vi "LINC Common Command Handler.vi"(6 "GUID":string, 8 "error in (no error)":errorcluster, 9 "command data in":string, 10 "command name in":string, 11 "LINC session":refnum<class "LINC.lvclass">) -> (0 "error out":errorcluster, 2 "application command":bool, 3 "dup LINC session":refnum<class "LINC.lvclass">)   [LabVIEW 2018, in "STEPkgDriver_LINC.lvlib" / "LINC.lvclass"]
uses:
  LINC.lvclass
  STEPkgDriver_LINC.lvlib
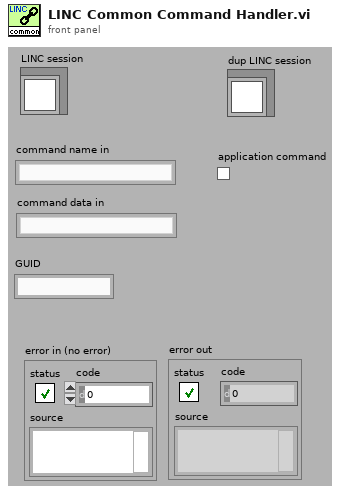
[diagram p1: front panel]
types:
  T1 = enum32{"Invalid", "Standard", "Closed", "Hidden", "Minimized", "Maximized"}
  T2 = cluster{"vi":string, "control":string, "value":variant}
  T3 = cluster{"mode (NO_SIM)":enum16{"NO_SIM", "SIM_EN", "SIM_DS"}, "defer update (F)":bool}
  T4 = typedef "LVRectTypeDef.ctl" = cluster{"Left":i16, "Top":i16, "Right":i16, "Bottom":i16}
  T5 = cluster{"VI":string, "CONTROL":string, "I16":i16}
  T6 = cluster{"VI":string, "CONTROL":string, "I32":i32}
  T7 = cluster{"VI":string, "CONTROL":string, "I64":i64}
  T8 = cluster{"VI":string, "CONTROL":string, "U16":u16}
  T9 = cluster{"VI":string, "CONTROL":string, "U32":u32}
  T10 = cluster{"VI":string, "CONTROL":string, "U64":u64}
  T11 = cluster{"VI":string, "CONTROL":string, "SGL":sgl}
  T12 = cluster{"VI":string, "CONTROL":string, "DBL":dbl}
  T13 = cluster{"VI":string, "CONTROL":string, "BOOL":bool}
  T14 = cluster{"VI":string, "CONTROL":string, "STR":string}
  T15 = cluster{"VI":string, "CONTROL":string, "PATH":string}
  T16 = cluster{"PACKET":string, "ITEM":string, "ST":bool, "VAL":i8}
  T17 = cluster{"PACKET":string, "ITEM":string, "ST":bool, "VAL":i16}
  T18 = cluster{"PACKET":string, "ITEM":string, "ST":bool, "VAL":i32}
  T19 = cluster{"PACKET":string, "ITEM":string, "ST":bool, "VAL":i64}
  T20 = cluster{"PACKET":string, "ITEM":string, "ST":bool, "VAL":u8}
  T21 = cluster{"PACKET":string, "ITEM":string, "ST":bool, "VAL":u16}
  T22 = cluster{"PACKET":string, "ITEM":string, "ST":bool, "VAL":u32}
  T23 = cluster{"PACKET":string, "ITEM":string, "ST":bool, "VAL":u64}
  T24 = cluster{"PACKET":string, "ITEM":string, "ST":bool, "VAL":sgl}
  T25 = cluster{"PACKET":string, "ITEM":string, "ST":bool, "VAL":dbl}
  T26 = cluster{"PACKET":string, "ITEM":string, "ST":bool, "VAL":bool}
  T27 = cluster{"PACKET":string, "ITEM":string, "ST":bool, "VAL":string}
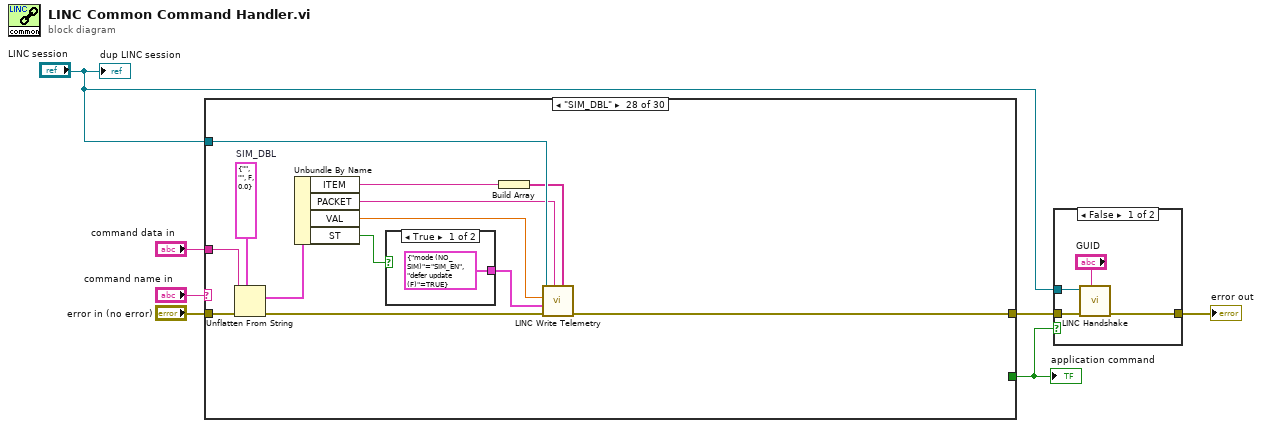
[diagram p0: block diagram]
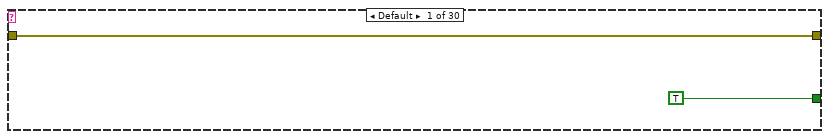
[diagram p3: hidden frame]
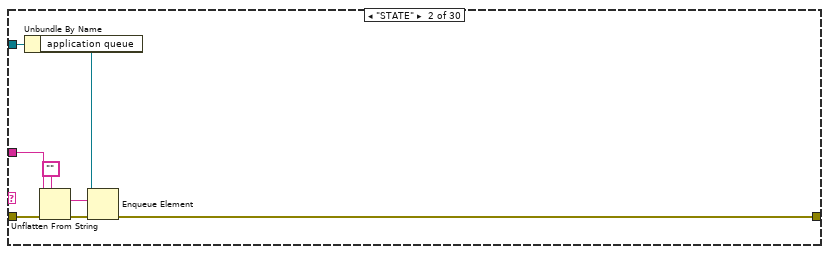
[diagram p4: hidden frame]
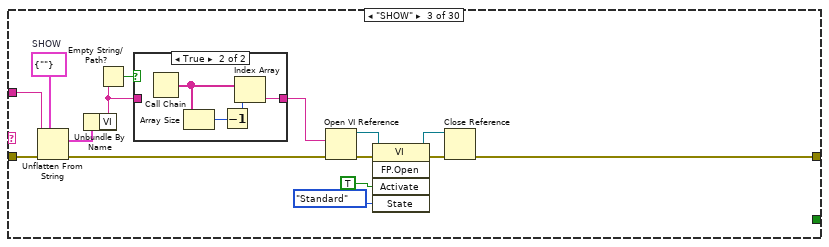
[diagram p5: hidden frame]
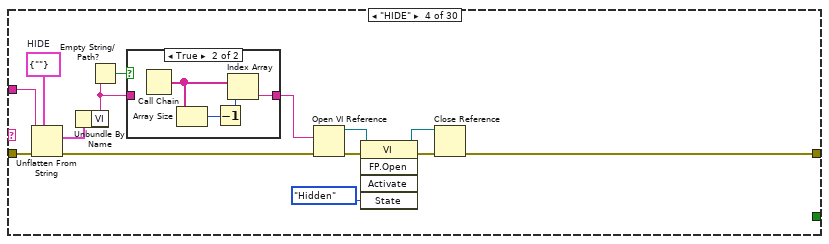
[diagram p7: hidden frame]
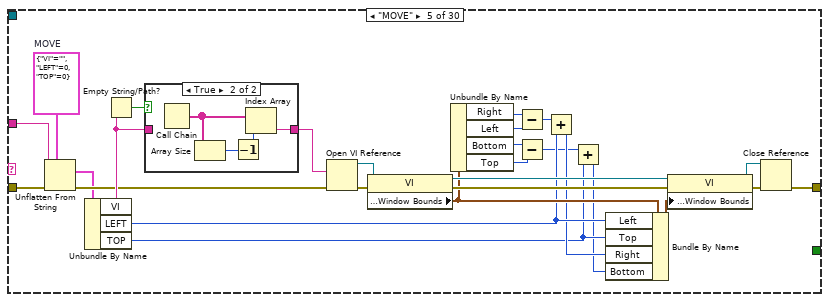
[diagram p9: hidden frame]
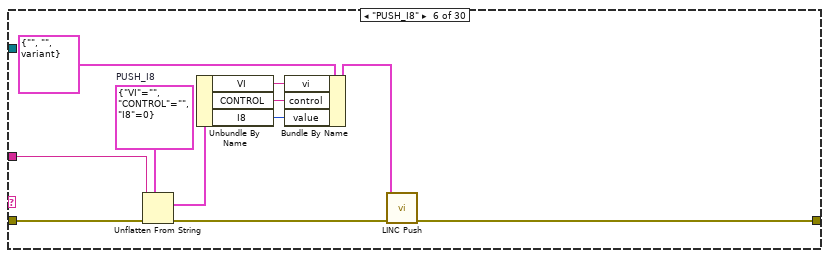
[diagram p11: hidden frame]
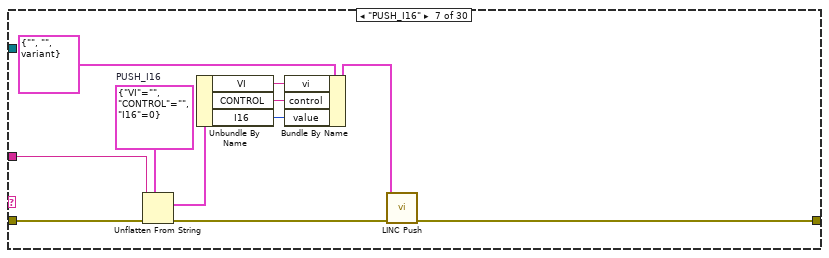
[diagram p12: hidden frame]
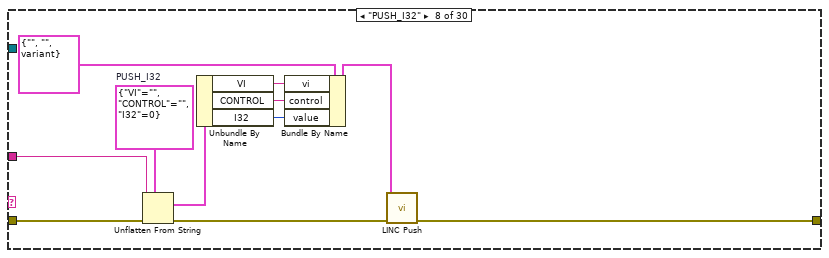
[diagram p13: hidden frame]
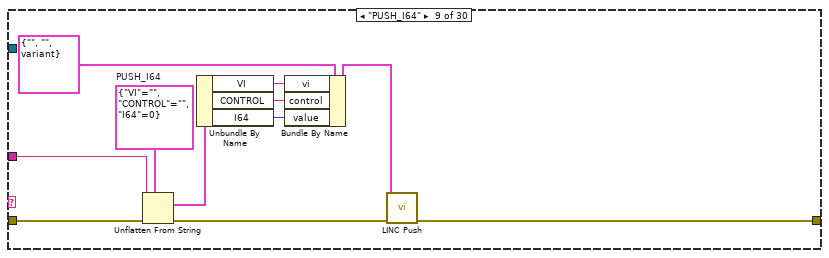
[diagram p14: hidden frame]
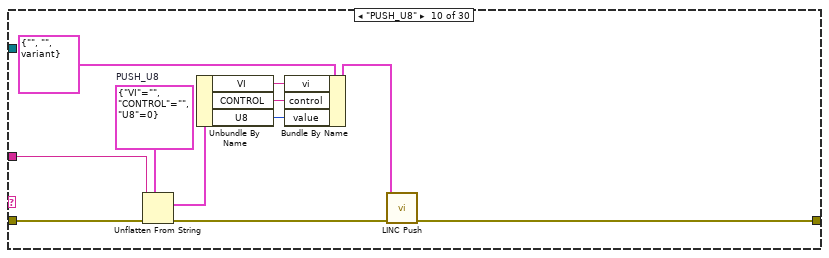
[diagram p15: hidden frame]
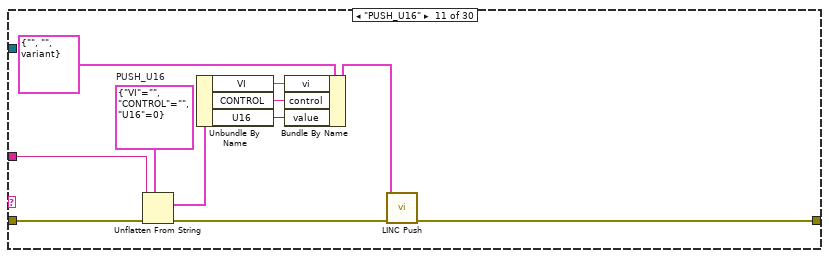
[diagram p16: hidden frame]
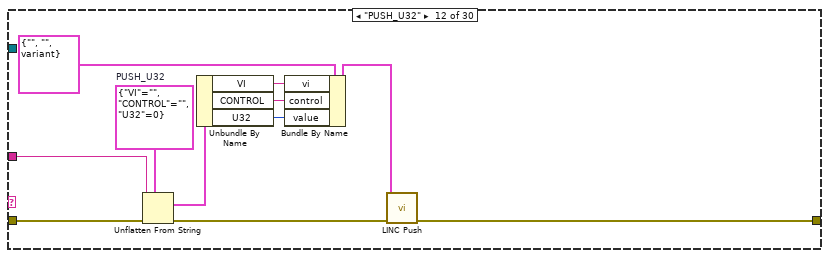
[diagram p17: hidden frame]
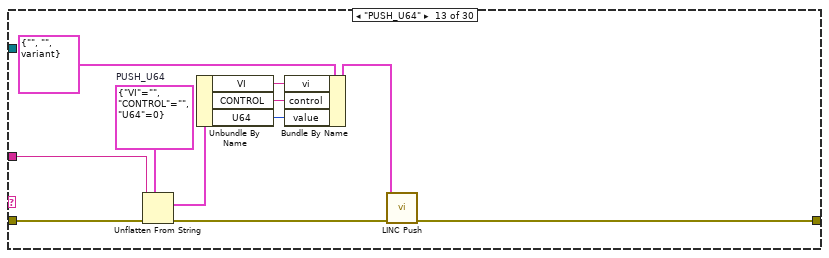
[diagram p18: hidden frame]
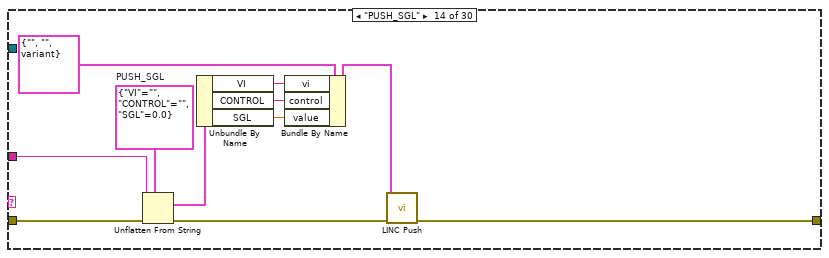
[diagram p19: hidden frame]
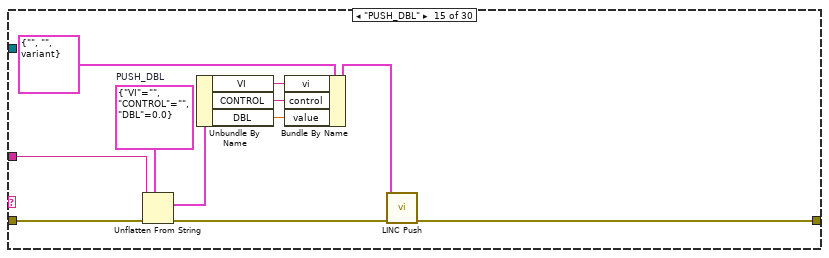
[diagram p20: hidden frame]
diagram:
  n1 = case shown="\"SIM_DBL\"" "command name in" {
    tunnel: "error in (no error)" -> [w9 w10 w25 w45 w61 w97 w108 w119 w130 w141 w152 w163 w174 w185 w196 w207 w218 w230 w244 w259 w274 w289 w304 w319 w334 w349 w364 w379 w394 w409]
    tunnel: [w9 w17 w32 w48 w82 w95 w106 w117 w128 w139 w150 w161 w172 w183 w194 w205 w216 w228 w240 w255 w270 w285 w300 w315 w330 w345 w360 w375 w390 w405] -> w4
    tunnel: "command data in" -> [_ w12 w24 w42 w60 w99 w110 w121 w132 w143 w154 w165 w176 w187 w198 w209 w220 w232 w245 w260 w275 w290 w305 w320 w335 w350 w365 w380 w395 w410]
    tunnel: [TRUE _ _ _ _ _ _ _ _ _ _ _ _ _ _ _ _ _ _ _ _ _ _ _ _ _ _ _ _ _] -> w3
    tunnel: "LINC session" -> [_ w13 _ _ _ _ _ _ _ _ _ _ _ _ _ _ _ _ w239 w254 w269 w284 w299 w314 w329 w344 w359 w374 w389 w404]
    frame Default {
    }
    frame "STATE" {
      n2 = Unbundle By Name(w13) -> ("application queue"=w11:refnum<queue>)
      n3 = Unflatten From String(type="", binary string=w12, error in (no error)=w10) -> (value=w14:string, error out=w16:errorcluster)  [unwired: 2 in, 1 out]
      n4 = Enqueue Element(queue=w11, element=w14, error in (no error)=w16) -> (error out=w17:errorcluster)  [unwired: 1 in, 2 out]
    }
    frame "SHOW" {
      w22 = cluster{"VI":string} {"VI"=""}  # SHOW
      n5 = Unflatten From String(type=w22, binary string=w24, error in (no error)=w25) -> (value=w21:cluster{"VI":string}, error out=w23:errorcluster)  [unwired: 2 in, 1 out]
      n6 = Unbundle By Name(w21) -> ("VI"=w19:string)
      n7 = Empty String/Path?(string/path=w19) -> (empty?=w20:bool)
      n8 = case shown="True" w20 {
        tunnel: [w33 w37] -> w18
        tunnel: w19 -> [w33 _]
        frame False {
        }
        frame True {
          n9 = Call Chain() -> (call chain=w36:string[])
          n10 = Array Size(array=w36) -> (size(s)=w35:i32)
          n11 = Decrement(x=w35) -> (x-1=w34:i32)
          n12 = Index Array(array=w36, index=w34) -> (element=w37:string)
        }
      }
      n13 = Open VI Reference(vi path=w18, error in (no error)=w23) -> (vi reference=w27:refnum<vi>, error out=w30:errorcluster)  [unwired: 4 in]
      n14 = invoke class="VI" method="FP.Open"(reference=w27, error in=w30, "Activate"=TRUE, "State"=T1."Standard") -> (reference out=w28:refnum<vi>, error out=w29:errorcluster)  [unwired: 1 in, 3 out]
      n15 = Close Reference(reference=w28, error in (no error)=w29) -> (error out=w32:errorcluster)
    }
    frame "HIDE" {
      w43 = cluster{"VI":string} {"VI"=""}  # HIDE
      n16 = Unflatten From String(type=w43, binary string=w42, error in (no error)=w45) -> (value=w41:cluster{"VI":string}, error out=w44:errorcluster)  [unwired: 2 in, 1 out]
      n17 = Unbundle By Name(w41) -> ("VI"=w39:string)
      n18 = Empty String/Path?(string/path=w39) -> (empty?=w40:bool)
      n19 = case shown="True" w40 {
        tunnel: [w52 w56] -> w38
        tunnel: w39 -> [w52 _]
        frame False {
        }
        frame True {
          n20 = Call Chain() -> (call chain=w55:string[])
          n21 = Array Size(array=w55) -> (size(s)=w54:i32)
          n22 = Decrement(x=w54) -> (x-1=w53:i32)
          n23 = Index Array(array=w55, index=w53) -> (element=w56:string)
        }
      }
      n24 = Open VI Reference(vi path=w38, error in (no error)=w44) -> (vi reference=w47:refnum<vi>, error out=w51:errorcluster)  [unwired: 4 in]
      n25 = invoke class="VI" method="FP.Open"(reference=w47, error in=w51, "State"=T1."Hidden") -> (reference out=w49:refnum<vi>, error out=w50:errorcluster)  [unwired: 2 in, 3 out]
      n26 = Close Reference(reference=w49, error in (no error)=w50) -> (error out=w48:errorcluster)
    }
    frame "MOVE" {
      w58 = cluster{"VI":string, "LEFT":i16, "TOP":i16} {"VI"="", "LEFT"=0, "TOP"=0}  # MOVE
      n27 = Unflatten From String(type=w58, binary string=w60, error in (no error)=w61) -> (value=w57:cluster{"VI":string, "LEFT":i16, "TOP":i16}, error out=w59:errorcluster)  [unwired: 2 in, 1 out]
      n28 = Unbundle By Name(w57) -> ("VI"=w80:string, "LEFT"=w69:i16, "TOP"=w66:i16)
      n29 = Empty String/Path?(string/path=w80) -> (empty?=w79:bool)
      n30 = case shown="True" w79 {
        tunnel: [w84 w88] -> w81
        tunnel: w80 -> [w84 _]
        frame False {
        }
        frame True {
          n31 = Call Chain() -> (call chain=w87:string[])
          n32 = Array Size(array=w87) -> (size(s)=w86:i32)
          n33 = Decrement(x=w86) -> (x-1=w85:i32)
          n34 = Index Array(array=w87, index=w85) -> (element=w88:string)
        }
      }
      n35 = Open VI Reference(vi path=w81, error in (no error)=w59) -> (vi reference=w75:refnum<vi>, error out=w77:errorcluster)  [unwired: 4 in]
      n36 = property class="VI"(reference=w75, error in=w77) -> (reference out=w74:refnum<vi>, error out=w76:errorcluster, "Front Panel Window:Window Bounds"=w71:T4)
      n37 = Unbundle By Name(w71) -> ("Right"=w73:i16, "Left"=w72:i16, "Bottom"=w64:i16, "Top"=w63:i16)
      n38 = Subtract(x=w73, y=w72) -> (x-y=w67:i16)
      n39 = Subtract(x=w64, y=w63) -> (x-y=w62:i16)
      n40 = Add(x=w67, y=w69) -> (x+y=w68:i16)
      n41 = Add(x=w62, y=w66) -> (x+y=w65:i16)
      n42 = Bundle By Name(cluster=w71, "Left"=w69, "Top"=w66, "Right"=w68, "Bottom"=w65) -> (w70:T4)
      n43 = property class="VI"(reference=w74, error in=w76, "Front Panel Window:Window Bounds"=w70) -> (reference out=w83:refnum<vi>, error out=w78:errorcluster)
      n44 = Close Reference(reference=w83, error in (no error)=w78) -> (error out=w82:errorcluster)
    }
    frame "PUSH_I8" {
      w93 = cluster{"VI":string, "CONTROL":string, "I8":i8} {"VI"="", "CONTROL"="", "I8"=0}  # PUSH_I8
      n45 = Unflatten From String(type=w93, binary string=w99, error in (no error)=w97) -> (value=w92:cluster{"VI":string, "CONTROL":string, "I8":i8}, error out=w96:errorcluster)  [unwired: 2 in, 1 out]
      n46 = Unbundle By Name(w92) -> ("VI"=w91:string, "CONTROL"=w90:string, "I8"=w89:i8)
      n47 = Bundle By Name(cluster=T2 {"vi"="", "control"="", "value"=variant}, "vi"=w91, "control"=w90, "value"=w89) -> (w94:T2)
      n48 = call "LINC Push.vi"("error in (no error)"=w96, "parameters"=w94) -> ("error out"=w95:errorcluster)  [unwired: 9 in]
    }
    frame "PUSH_I16" {
      w104 = T5 {"VI"="", "CONTROL"="", "I16"=0}  # PUSH_I16
      n49 = Unflatten From String(type=w104, binary string=w110, error in (no error)=w108) -> (value=w103:T5, error out=w107:errorcluster)  [unwired: 2 in, 1 out]
      n50 = Unbundle By Name(w103) -> ("VI"=w102:string, "CONTROL"=w101:string, "I16"=w100:i16)
      n51 = Bundle By Name(cluster=T2 {"vi"="", "control"="", "value"=variant}, "vi"=w102, "control"=w101, "value"=w100) -> (w105:T2)
      n52 = call "LINC Push.vi"("error in (no error)"=w107, "parameters"=w105) -> ("error out"=w106:errorcluster)  [unwired: 9 in]
    }
    frame "PUSH_I32" {
      w115 = T6 {"VI"="", "CONTROL"="", "I32"=0}  # PUSH_I32
      n53 = Unflatten From String(type=w115, binary string=w121, error in (no error)=w119) -> (value=w114:T6, error out=w118:errorcluster)  [unwired: 2 in, 1 out]
      n54 = Unbundle By Name(w114) -> ("VI"=w113:string, "CONTROL"=w112:string, "I32"=w111:i32)
      n55 = Bundle By Name(cluster=T2 {"vi"="", "control"="", "value"=variant}, "vi"=w113, "control"=w112, "value"=w111) -> (w116:T2)
      n56 = call "LINC Push.vi"("error in (no error)"=w118, "parameters"=w116) -> ("error out"=w117:errorcluster)  [unwired: 9 in]
    }
    frame "PUSH_I64" {
      w126 = T7 {"VI"="", "CONTROL"="", "I64"=0}  # PUSH_I64
      n57 = Unflatten From String(type=w126, binary string=w132, error in (no error)=w130) -> (value=w125:T7, error out=w129:errorcluster)  [unwired: 2 in, 1 out]
      n58 = Unbundle By Name(w125) -> ("VI"=w124:string, "CONTROL"=w123:string, "I64"=w122:i64)
      n59 = Bundle By Name(cluster=T2 {"vi"="", "control"="", "value"=variant}, "vi"=w124, "control"=w123, "value"=w122) -> (w127:T2)
      n60 = call "LINC Push.vi"("error in (no error)"=w129, "parameters"=w127) -> ("error out"=w128:errorcluster)  [unwired: 9 in]
    }
    frame "PUSH_U8" {
      w137 = cluster{"VI":string, "CONTROL":string, "U8":u8} {"VI"="", "CONTROL"="", "U8"=0}  # PUSH_U8
      n61 = Unflatten From String(type=w137, binary string=w143, error in (no error)=w141) -> (value=w136:cluster{"VI":string, "CONTROL":string, "U8":u8}, error out=w140:errorcluster)  [unwired: 2 in, 1 out]
      n62 = Unbundle By Name(w136) -> ("VI"=w135:string, "CONTROL"=w134:string, "U8"=w133:u8)
      n63 = Bundle By Name(cluster=T2 {"vi"="", "control"="", "value"=variant}, "vi"=w135, "control"=w134, "value"=w133) -> (w138:T2)
      n64 = call "LINC Push.vi"("error in (no error)"=w140, "parameters"=w138) -> ("error out"=w139:errorcluster)  [unwired: 9 in]
    }
    frame "PUSH_U16" {
      w148 = T8 {"VI"="", "CONTROL"="", "U16"=0}  # PUSH_U16
      n65 = Unflatten From String(type=w148, binary string=w154, error in (no error)=w152) -> (value=w147:T8, error out=w151:errorcluster)  [unwired: 2 in, 1 out]
      n66 = Unbundle By Name(w147) -> ("VI"=w146:string, "CONTROL"=w145:string, "U16"=w144:u16)
      n67 = Bundle By Name(cluster=T2 {"vi"="", "control"="", "value"=variant}, "vi"=w146, "control"=w145, "value"=w144) -> (w149:T2)
      n68 = call "LINC Push.vi"("error in (no error)"=w151, "parameters"=w149) -> ("error out"=w150:errorcluster)  [unwired: 9 in]
    }
    frame "PUSH_U32" {
      w159 = T9 {"VI"="", "CONTROL"="", "U32"=0}  # PUSH_U32
      n69 = Unflatten From String(type=w159, binary string=w165, error in (no error)=w163) -> (value=w158:T9, error out=w162:errorcluster)  [unwired: 2 in, 1 out]
      n70 = Unbundle By Name(w158) -> ("VI"=w157:string, "CONTROL"=w156:string, "U32"=w155:u32)
      n71 = Bundle By Name(cluster=T2 {"vi"="", "control"="", "value"=variant}, "vi"=w157, "control"=w156, "value"=w155) -> (w160:T2)
      n72 = call "LINC Push.vi"("error in (no error)"=w162, "parameters"=w160) -> ("error out"=w161:errorcluster)  [unwired: 9 in]
    }
    frame "PUSH_U64" {
      w170 = T10 {"VI"="", "CONTROL"="", "U64"=0}  # PUSH_U64
      n73 = Unflatten From String(type=w170, binary string=w176, error in (no error)=w174) -> (value=w169:T10, error out=w173:errorcluster)  [unwired: 2 in, 1 out]
      n74 = Unbundle By Name(w169) -> ("VI"=w168:string, "CONTROL"=w167:string, "U64"=w166:u64)
      n75 = Bundle By Name(cluster=T2 {"vi"="", "control"="", "value"=variant}, "vi"=w168, "control"=w167, "value"=w166) -> (w171:T2)
      n76 = call "LINC Push.vi"("error in (no error)"=w173, "parameters"=w171) -> ("error out"=w172:errorcluster)  [unwired: 9 in]
    }
    frame "PUSH_SGL" {
      w181 = T11 {"VI"="", "CONTROL"="", "SGL"=0.0}  # PUSH_SGL
      n77 = Unflatten From String(type=w181, binary string=w187, error in (no error)=w185) -> (value=w180:T11, error out=w184:errorcluster)  [unwired: 2 in, 1 out]
      n78 = Unbundle By Name(w180) -> ("VI"=w179:string, "CONTROL"=w178:string, "SGL"=w177:sgl)
      n79 = Bundle By Name(cluster=T2 {"vi"="", "control"="", "value"=variant}, "vi"=w179, "control"=w178, "value"=w177) -> (w182:T2)
      n80 = call "LINC Push.vi"("error in (no error)"=w184, "parameters"=w182) -> ("error out"=w183:errorcluster)  [unwired: 9 in]
    }
    frame "PUSH_DBL" {
      w192 = T12 {"VI"="", "CONTROL"="", "DBL"=0.0}  # PUSH_DBL
      n81 = Unflatten From String(type=w192, binary string=w198, error in (no error)=w196) -> (value=w191:T12, error out=w195:errorcluster)  [unwired: 2 in, 1 out]
      n82 = Unbundle By Name(w191) -> ("VI"=w190:string, "CONTROL"=w189:string, "DBL"=w188:dbl)
      n83 = Bundle By Name(cluster=T2 {"vi"="", "control"="", "value"=variant}, "vi"=w190, "control"=w189, "value"=w188) -> (w193:T2)
      n84 = call "LINC Push.vi"("error in (no error)"=w195, "parameters"=w193) -> ("error out"=w194:errorcluster)  [unwired: 9 in]
    }
    frame "PUSH_BOOL" {
      w203 = T13 {"VI"="", "CONTROL"="", "BOOL"=FALSE}  # PUSH_BOOL
      n85 = Unflatten From String(type=w203, binary string=w209, error in (no error)=w207) -> (value=w202:T13, error out=w206:errorcluster)  [unwired: 2 in, 1 out]
      n86 = Unbundle By Name(w202) -> ("VI"=w201:string, "CONTROL"=w200:string, "BOOL"=w199:bool)
      n87 = Bundle By Name(cluster=T2 {"vi"="", "control"="", "value"=variant}, "vi"=w201, "control"=w200, "value"=w199) -> (w204:T2)
      n88 = call "LINC Push.vi"("error in (no error)"=w206, "parameters"=w204) -> ("error out"=w205:errorcluster)  [unwired: 9 in]
    }
    frame "PUSH_STR" {
      w214 = T14 {"VI"="", "CONTROL"="", "STR"=""}  # PUSH_STR
      n89 = Unflatten From String(type=w214, binary string=w220, error in (no error)=w218) -> (value=w213:T14, error out=w217:errorcluster)  [unwired: 2 in, 1 out]
      n90 = Unbundle By Name(w213) -> ("VI"=w212:string, "CONTROL"=w211:string, "STR"=w210:string)
      n91 = Bundle By Name(cluster=T2 {"vi"="", "control"="", "value"=variant}, "vi"=w212, "control"=w211, "value"=w210) -> (w215:T2)
      n92 = call "LINC Push.vi"("error in (no error)"=w217, "parameters"=w215) -> ("error out"=w216:errorcluster)  [unwired: 9 in]
    }
    frame "PUSH_PATH" {
      w226 = T15 {"VI"="", "CONTROL"="", "PATH"=""}  # PUSH_PATH
      n93 = Unflatten From String(type=w226, binary string=w232, error in (no error)=w230) -> (value=w225:T15, error out=w229:errorcluster)  [unwired: 2 in, 1 out]
      n94 = Unbundle By Name(w225) -> ("VI"=w224:string, "CONTROL"=w223:string, "PATH"=w222:string)
      n95 = String To Path(string=w222) -> (path=w221:path)
      n96 = Bundle By Name(cluster=T2 {"vi"="", "control"="", "value"=variant}, "vi"=w224, "control"=w223, "value"=w221) -> (w227:T2)
      n97 = call "LINC Push.vi"("error in (no error)"=w229, "parameters"=w227) -> ("error out"=w228:errorcluster)  [unwired: 9 in]
    }
    frame "SIM_I8" {
      w242 = T16 {"PACKET"="", "ITEM"="", "ST"=FALSE, "VAL"=0}  # SIM_I8
      n98 = Unflatten From String(type=w242, binary string=w245, error in (no error)=w244) -> (value=w243:T16, error out=w241:errorcluster)  [unwired: 2 in, 1 out]
      n99 = Unbundle By Name(w243) -> ("ITEM"=w236:string, "PACKET"=w238:string, "VAL"=w237:i8, "ST"=w234:bool)
      n100 = case shown="True" w234 {
        tunnel: [T3 {"mode (NO_SIM)"=enum."SIM_EN", "defer update (F)"=TRUE} ("options") T3 {"mode (NO_SIM)"=enum."SIM_DS", "defer update (F)"=TRUE} ("options")] -> w233
        frame True {
        }
        frame False {
        }
      }
      n101 = Build Array(w236) -> (w235:string[])
      n102 = call "LINC Write Telemetry.vi"("data names"=w235, "packet name"=w238, "error in (no error)"=w241, "options"=w233, "packet"=w237, "LINC session"=w239) -> ("error out"=w240:errorcluster)  [unwired: 4 in, 1 out]
    }
    frame "SIM_I16" {
      w257 = T17 {"PACKET"="", "ITEM"="", "ST"=FALSE, "VAL"=0}  # SIM_I16
      n103 = Unflatten From String(type=w257, binary string=w260, error in (no error)=w259) -> (value=w258:T17, error out=w256:errorcluster)  [unwired: 2 in, 1 out]
      n104 = Unbundle By Name(w258) -> ("ITEM"=w251:string, "PACKET"=w253:string, "VAL"=w252:i16, "ST"=w249:bool)
      n105 = case shown="True" w249 {
        tunnel: [T3 {"mode (NO_SIM)"=enum."SIM_EN", "defer update (F)"=TRUE} ("options") T3 {"mode (NO_SIM)"=enum."SIM_DS", "defer update (F)"=TRUE} ("options")] -> w248
        frame True {
        }
        frame False {
        }
      }
      n106 = Build Array(w251) -> (w250:string[])
      n107 = call "LINC Write Telemetry.vi"("data names"=w250, "packet name"=w253, "error in (no error)"=w256, "options"=w248, "packet"=w252, "LINC session"=w254) -> ("error out"=w255:errorcluster)  [unwired: 4 in, 1 out]
    }
    frame "SIM_I32" {
      w272 = T18 {"PACKET"="", "ITEM"="", "ST"=FALSE, "VAL"=0}  # SIM_I32
      n108 = Unflatten From String(type=w272, binary string=w275, error in (no error)=w274) -> (value=w273:T18, error out=w271:errorcluster)  [unwired: 2 in, 1 out]
      n109 = Unbundle By Name(w273) -> ("ITEM"=w266:string, "PACKET"=w268:string, "VAL"=w267:i32, "ST"=w264:bool)
      n110 = case shown="True" w264 {
        tunnel: [T3 {"mode (NO_SIM)"=enum."SIM_EN", "defer update (F)"=TRUE} ("options") T3 {"mode (NO_SIM)"=enum."SIM_DS", "defer update (F)"=TRUE} ("options")] -> w263
        frame True {
        }
        frame False {
        }
      }
      n111 = Build Array(w266) -> (w265:string[])
      n112 = call "LINC Write Telemetry.vi"("data names"=w265, "packet name"=w268, "error in (no error)"=w271, "options"=w263, "packet"=w267, "LINC session"=w269) -> ("error out"=w270:errorcluster)  [unwired: 4 in, 1 out]
    }
    frame "SIM_I64" {
      w287 = T19 {"PACKET"="", "ITEM"="", "ST"=FALSE, "VAL"=0}  # SIM_I64
      n113 = Unflatten From String(type=w287, binary string=w290, error in (no error)=w289) -> (value=w288:T19, error out=w286:errorcluster)  [unwired: 2 in, 1 out]
      n114 = Unbundle By Name(w288) -> ("ITEM"=w281:string, "PACKET"=w283:string, "VAL"=w282:i64, "ST"=w279:bool)
      n115 = case shown="True" w279 {
        tunnel: [T3 {"mode (NO_SIM)"=enum."SIM_EN", "defer update (F)"=TRUE} ("options") T3 {"mode (NO_SIM)"=enum."SIM_DS", "defer update (F)"=TRUE} ("options")] -> w278
        frame True {
        }
        frame False {
        }
      }
      n116 = Build Array(w281) -> (w280:string[])
      n117 = call "LINC Write Telemetry.vi"("data names"=w280, "packet name"=w283, "error in (no error)"=w286, "options"=w278, "packet"=w282, "LINC session"=w284) -> ("error out"=w285:errorcluster)  [unwired: 4 in, 1 out]
    }
    frame "SIM_U8" {
      w302 = T20 {"PACKET"="", "ITEM"="", "ST"=FALSE, "VAL"=0}  # SIM_U8
      n118 = Unflatten From String(type=w302, binary string=w305, error in (no error)=w304) -> (value=w303:T20, error out=w301:errorcluster)  [unwired: 2 in, 1 out]
      n119 = Unbundle By Name(w303) -> ("ITEM"=w296:string, "PACKET"=w298:string, "VAL"=w297:u8, "ST"=w294:bool)
      n120 = case shown="True" w294 {
        tunnel: [T3 {"mode (NO_SIM)"=enum."SIM_EN", "defer update (F)"=TRUE} ("options") T3 {"mode (NO_SIM)"=enum."SIM_DS", "defer update (F)"=TRUE} ("options")] -> w293
        frame True {
        }
        frame False {
        }
      }
      n121 = Build Array(w296) -> (w295:string[])
      n122 = call "LINC Write Telemetry.vi"("data names"=w295, "packet name"=w298, "error in (no error)"=w301, "options"=w293, "packet"=w297, "LINC session"=w299) -> ("error out"=w300:errorcluster)  [unwired: 4 in, 1 out]
    }
    frame "SIM_U16" {
      w317 = T21 {"PACKET"="", "ITEM"="", "ST"=FALSE, "VAL"=0}  # SIM_U16
      n123 = Unflatten From String(type=w317, binary string=w320, error in (no error)=w319) -> (value=w318:T21, error out=w316:errorcluster)  [unwired: 2 in, 1 out]
      n124 = Unbundle By Name(w318) -> ("ITEM"=w311:string, "PACKET"=w313:string, "VAL"=w312:u16, "ST"=w309:bool)
      n125 = case shown="True" w309 {
        tunnel: [T3 {"mode (NO_SIM)"=enum."SIM_EN", "defer update (F)"=TRUE} ("options") T3 {"mode (NO_SIM)"=enum."SIM_DS", "defer update (F)"=TRUE} ("options")] -> w308
        frame True {
        }
        frame False {
        }
      }
      n126 = Build Array(w311) -> (w310:string[])
      n127 = call "LINC Write Telemetry.vi"("data names"=w310, "packet name"=w313, "error in (no error)"=w316, "options"=w308, "packet"=w312, "LINC session"=w314) -> ("error out"=w315:errorcluster)  [unwired: 4 in, 1 out]
    }
    frame "SIM_U32" {
      w332 = T22 {"PACKET"="", "ITEM"="", "ST"=FALSE, "VAL"=0}  # SIM_U32
      n128 = Unflatten From String(type=w332, binary string=w335, error in (no error)=w334) -> (value=w333:T22, error out=w331:errorcluster)  [unwired: 2 in, 1 out]
      n129 = Unbundle By Name(w333) -> ("ITEM"=w326:string, "PACKET"=w328:string, "VAL"=w327:u32, "ST"=w324:bool)
      n130 = case shown="True" w324 {
        tunnel: [T3 {"mode (NO_SIM)"=enum."SIM_EN", "defer update (F)"=TRUE} ("options") T3 {"mode (NO_SIM)"=enum."SIM_DS", "defer update (F)"=TRUE} ("options")] -> w323
        frame True {
        }
        frame False {
        }
      }
      n131 = Build Array(w326) -> (w325:string[])
      n132 = call "LINC Write Telemetry.vi"("data names"=w325, "packet name"=w328, "error in (no error)"=w331, "options"=w323, "packet"=w327, "LINC session"=w329) -> ("error out"=w330:errorcluster)  [unwired: 4 in, 1 out]
    }
    frame "SIM_U64" {
      w347 = T23 {"PACKET"="", "ITEM"="", "ST"=FALSE, "VAL"=0}  # SIM_U64
      n133 = Unflatten From String(type=w347, binary string=w350, error in (no error)=w349) -> (value=w348:T23, error out=w346:errorcluster)  [unwired: 2 in, 1 out]
      n134 = Unbundle By Name(w348) -> ("ITEM"=w341:string, "PACKET"=w343:string, "VAL"=w342:u64, "ST"=w339:bool)
      n135 = case shown="True" w339 {
        tunnel: [T3 {"mode (NO_SIM)"=enum."SIM_EN", "defer update (F)"=TRUE} ("options") T3 {"mode (NO_SIM)"=enum."SIM_DS", "defer update (F)"=TRUE} ("options")] -> w338
        frame True {
        }
        frame False {
        }
      }
      n136 = Build Array(w341) -> (w340:string[])
      n137 = call "LINC Write Telemetry.vi"("data names"=w340, "packet name"=w343, "error in (no error)"=w346, "options"=w338, "packet"=w342, "LINC session"=w344) -> ("error out"=w345:errorcluster)  [unwired: 4 in, 1 out]
    }
    frame "SIM_SGL" {
      w362 = T24 {"PACKET"="", "ITEM"="", "ST"=FALSE, "VAL"=0.0}  # SIM_SGL
      n138 = Unflatten From String(type=w362, binary string=w365, error in (no error)=w364) -> (value=w363:T24, error out=w361:errorcluster)  [unwired: 2 in, 1 out]
      n139 = Unbundle By Name(w363) -> ("ITEM"=w356:string, "PACKET"=w358:string, "VAL"=w357:sgl, "ST"=w354:bool)
      n140 = case shown="True" w354 {
        tunnel: [T3 {"mode (NO_SIM)"=enum."SIM_EN", "defer update (F)"=TRUE} ("options") T3 {"mode (NO_SIM)"=enum."SIM_DS", "defer update (F)"=TRUE} ("options")] -> w353
        frame True {
        }
        frame False {
        }
      }
      n141 = Build Array(w356) -> (w355:string[])
      n142 = call "LINC Write Telemetry.vi"("data names"=w355, "packet name"=w358, "error in (no error)"=w361, "options"=w353, "packet"=w357, "LINC session"=w359) -> ("error out"=w360:errorcluster)  [unwired: 4 in, 1 out]
    }
    frame "SIM_DBL" {
      w377 = T25 {"PACKET"="", "ITEM"="", "ST"=FALSE, "VAL"=0.0}  # SIM_DBL
      n143 = Unflatten From String(type=w377, binary string=w380, error in (no error)=w379) -> (value=w378:T25, error out=w376:errorcluster)  [unwired: 2 in, 1 out]
      n144 = Unbundle By Name(w378) -> ("ITEM"=w371:string, "PACKET"=w373:string, "VAL"=w372:dbl, "ST"=w369:bool)
      n145 = case shown="True" w369 {
        tunnel: [T3 {"mode (NO_SIM)"=enum."SIM_EN", "defer update (F)"=TRUE} ("options") T3 {"mode (NO_SIM)"=enum."SIM_DS", "defer update (F)"=TRUE} ("options")] -> w368
        frame True {
        }
        frame False {
        }
      }
      n146 = Build Array(w371) -> (w370:string[])
      n147 = call "LINC Write Telemetry.vi"("data names"=w370, "packet name"=w373, "error in (no error)"=w376, "options"=w368, "packet"=w372, "LINC session"=w374) -> ("error out"=w375:errorcluster)  [unwired: 4 in, 1 out]
    }
    frame "SIM_BOOL" {
      w392 = T26 {"PACKET"="", "ITEM"="", "ST"=FALSE, "VAL"=FALSE}  # SIM_BOOL
      n148 = Unflatten From String(type=w392, binary string=w395, error in (no error)=w394) -> (value=w393:T26, error out=w391:errorcluster)  [unwired: 2 in, 1 out]
      n149 = Unbundle By Name(w393) -> ("ITEM"=w386:string, "PACKET"=w388:string, "VAL"=w387:bool, "ST"=w384:bool)
      n150 = case shown="True" w384 {
        tunnel: [T3 {"mode (NO_SIM)"=enum."SIM_EN", "defer update (F)"=TRUE} ("options") T3 {"mode (NO_SIM)"=enum."SIM_DS", "defer update (F)"=TRUE} ("options")] -> w383
        frame True {
        }
        frame False {
        }
      }
      n151 = Build Array(w386) -> (w385:string[])
      n152 = call "LINC Write Telemetry.vi"("data names"=w385, "packet name"=w388, "error in (no error)"=w391, "options"=w383, "packet"=w387, "LINC session"=w389) -> ("error out"=w390:errorcluster)  [unwired: 4 in, 1 out]
    }
    frame "SIM_STR" {
      w407 = T27 {"PACKET"="", "ITEM"="", "ST"=FALSE, "VAL"=""}  # SIM_STR
      n153 = Unflatten From String(type=w407, binary string=w410, error in (no error)=w409) -> (value=w408:T27, error out=w406:errorcluster)  [unwired: 2 in, 1 out]
      n154 = Unbundle By Name(w408) -> ("ITEM"=w401:string, "PACKET"=w403:string, "VAL"=w402:string, "ST"=w399:bool)
      n155 = case shown="True" w399 {
        tunnel: [T3 {"mode (NO_SIM)"=enum."SIM_EN", "defer update (F)"=TRUE} ("options") T3 {"mode (NO_SIM)"=enum."SIM_DS", "defer update (F)"=TRUE} ("options")] -> w398
        frame True {
        }
        frame False {
        }
      }
      n156 = Build Array(w401) -> (w400:string[])
      n157 = call "LINC Write Telemetry.vi"("data names"=w400, "packet name"=w403, "error in (no error)"=w406, "options"=w398, "packet"=w402, "LINC session"=w404) -> ("error out"=w405:errorcluster)  [unwired: 4 in, 1 out]
    }
  }
  "application command" <- w3
  n158 = case shown="False" w3 {
    tunnel: w4 -> [w416 w417]
    tunnel: [w415 w417] -> w2
    tunnel: "LINC session" -> [w414 _]
    frame False {
      n159 = call "LINC Handshake.vi"("GUID (optional)"="GUID", "error in (no error)"=w416, "LINC session"=w414) -> ("error out"=w415:errorcluster)  [unwired: 7 in, 1 out]
    }
    frame True {
    }
  }
  "error out" <- w2
  "dup LINC session" <- "LINC session"
